vi "Write Device Metadata.vi"(0 "File Path":path, 11 "Error In":errorcluster) -> (4 "File Path (Dup)":path, 15 "Error Out":errorcluster)   [LabVIEW 2020]
uses:
  Hardware Configuration/Hardware Configuration Controls/Device Type.ctl
  Device Library/AOTFs/AOTF Controls/AOTF Actions.ctl
  Device Library/Cameras/Camera Controls/Generic Camera Actions.ctl
  Device Library/Lasers/Laser Controls/Laser Actions.ctl
  Device Library/Shutters/Shutter Controls/Shutter Actions.ctl
  Device Library/Stages/Stages Controls/Stage Actions.ctl
  Device Library/Filter Wheels/Polymorphic Filter Wheel Messenger/FW Get Position.vi
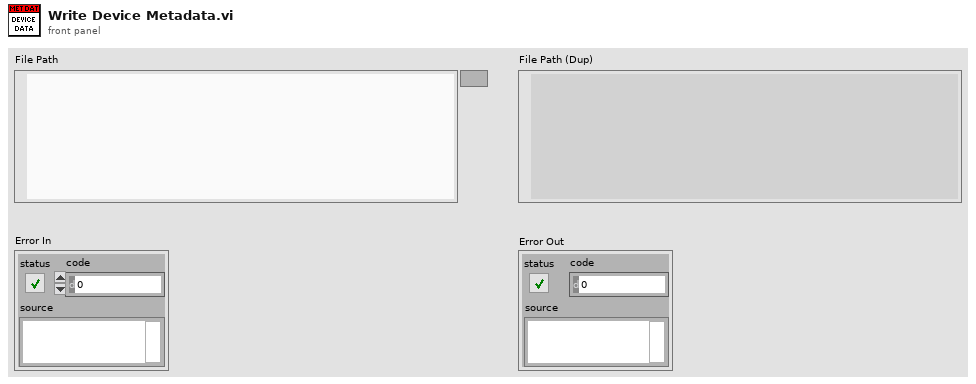
[diagram p1: front panel]
types:
  T1 = enum16{"open", "replace", "create", "open or create", "replace or create", "replace or create with confirmation"}
  T2 = typedef "Device Type.ctl" = enum16{"AOTF", "Camera", "Deformable Mirror", "Laser", "Microscope Base", "Shutter", "Stage", "Waveform", "FPGA", "Email", "Filter Wheel", "Spinning Disk"}
  T3 = typedef "Generic Camera Actions.ctl" = enum16{"Status", "Live Preview", "Capture", "Abort", "Set Exposure Time (s)", "Get Exposure Time (s)", "Record Settings", "Binning", "Set ROI", "Get ROI", "Defect Correction On?", "Cooler On?", "Fan On?", "Quit"}
  T4 = typedef "Laser Actions.ctl" = enum16{"Error Check", "Set On/Off", "Set Power", "Set Parameter", "Get Power", "Get Status", "Get Parameter", "Quit"}
  T5 = typedef "Shutter Actions.ctl" = enum16{"Open", "Close", "Toggle", "Status", "Quit"}
  T6 = typedef "Stage Actions.ctl" = enum16{"Get Position", "MVR", "MOVE", "HALT", "ONTARGET", "ERROR", "REFERENCE", "INIT", "VELOCITY", "STATUS", "EXIT", "HOME", "ZEROPOS", "NANOPOS", "ANALOG", "QUIT"}
  T7 = typedef "AOTF Actions.ctl" = enum16{"Error Check", "Blank", "Line On/Off", "Set Power", "Status", "Quit"}
  T8 = typedef "Laser Status.ctl" = enum16{"Warmup", "Ready", "Emission", "Tuning", "Error"}
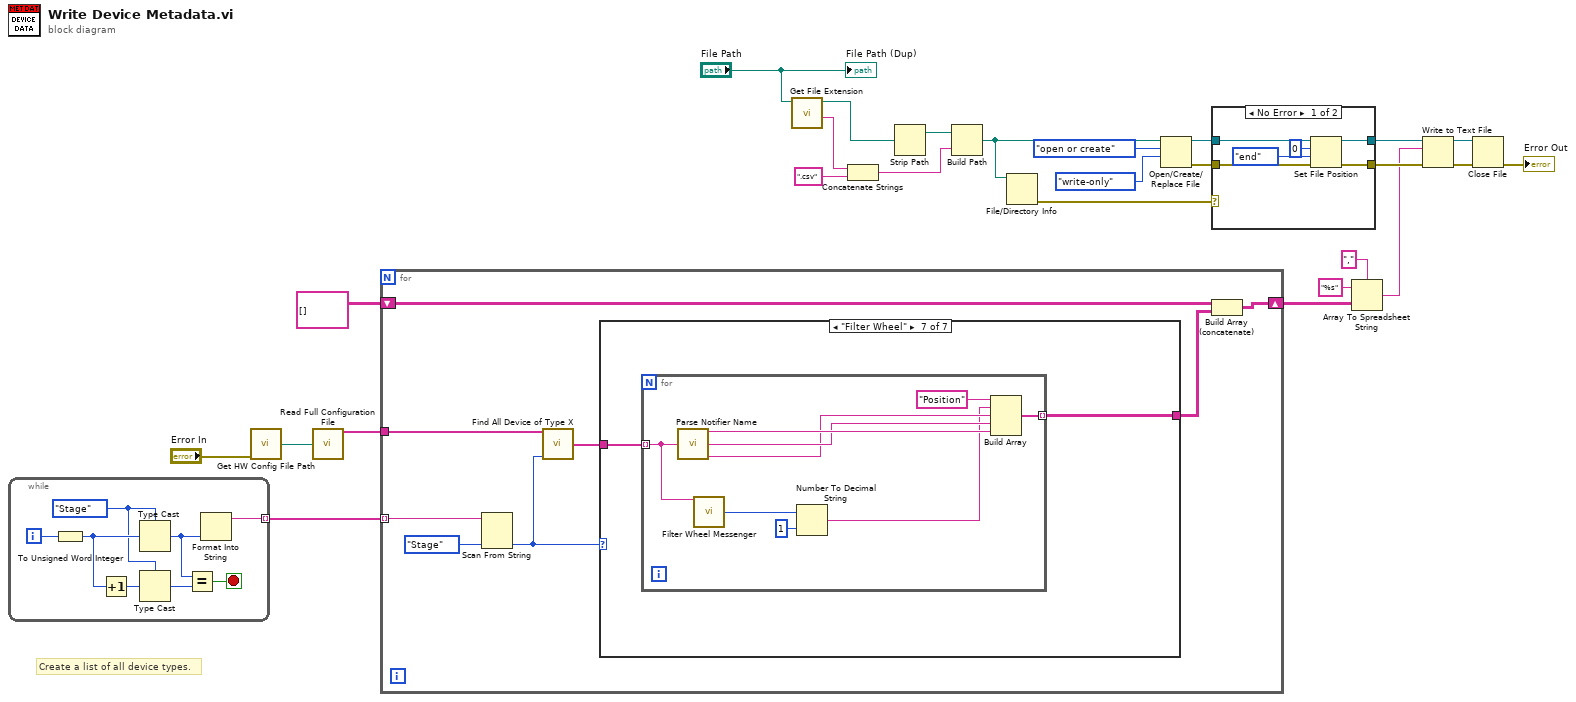
[diagram p0: block diagram]
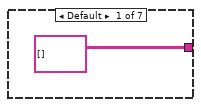
[diagram p3: hidden frame]
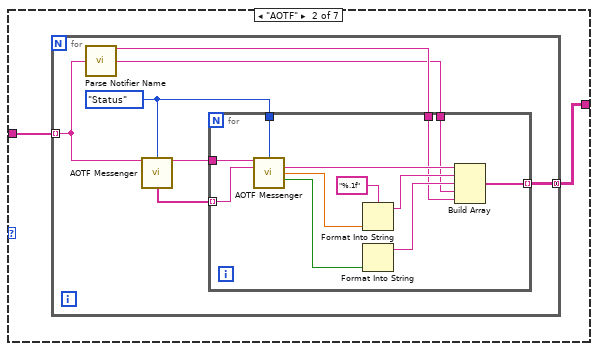
[diagram p4: hidden frame]
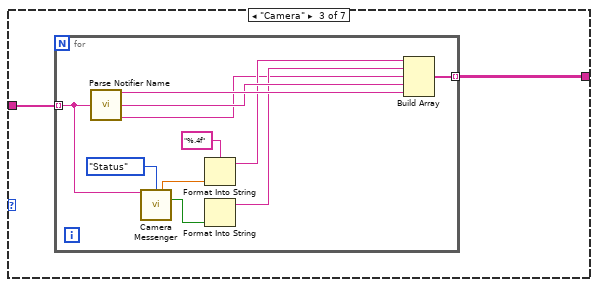
[diagram p5: hidden frame]
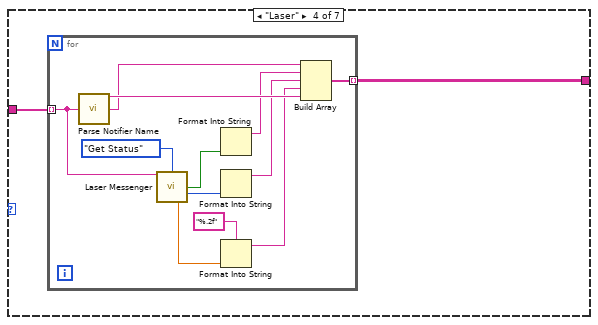
[diagram p6: hidden frame]
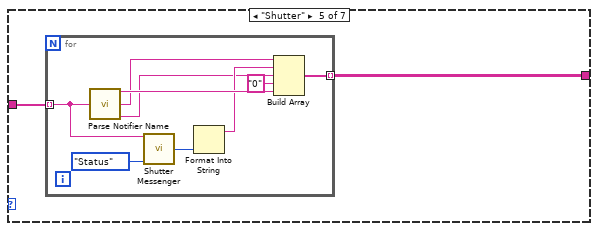
[diagram p7: hidden frame]
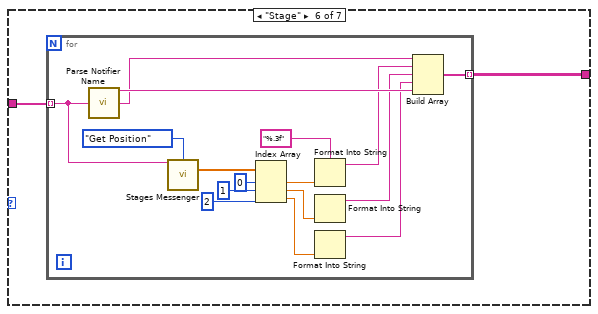
[diagram p8: hidden frame]
diagram:
  # "Create a list of all device types."
  n1 = while {
    tunnel: [w27] -> w26 mode=indexing
    i -> [w30]
    stop <- w29 stop-if-true
    w31 = Device_Type."Stage" ("Device Type")
    n2 = To Unsigned Word Integer(number=w30) -> (unsigned 16bit integer=w32:u16)
    n3 = Increment(x=w32) -> (x+1=w33:u16)
    n4 = Type Cast(type=w31, x=w32) -> (*(type *) &x=w28:T2)
    n5 = Type Cast(type=w31, x=w33) -> (*(type *) &x=w34:T2)
    n6 = Equal?(x=w28, y=w34) -> (x = y?=w29:bool)
    n7 = Format Into String(w28) -> (resulting string=w27:string)  [unwired: 3 in, 1 out]
  }
  n8 = call "Get HW Config File Path.vi"("Error"="Error In") -> ("File Path"=w25:path)  [unwired: 13 in, 1 out]
  n9 = call "Read Full Configuration File.vi"("Config File Path"=w25) -> ("Unique Notifier Names"=w24:string[])  [unwired: 11 in, 3 out]
  n10 = for {
    tunnel: w26 -> [w42] mode=indexing
    tunnel: w24 -> [w39]
    shift-right: [w36] -> w2
    shift-left: string[][] [] -> [w37]
    n11 = Scan From String(input string=w42, default 1=Device_Type."Stage" ("Device Type")) -> (output 1=w40:T2)  [unwired: 3 in, 3 out]
    n12 = call "Find All Device of Type X.vi"("Unique Notifier Names"=w39, "Device Type"=w40) -> ("Running Devices"=w38:string[])  [unwired: 12 in, 1 out]
    n13 = case shown="\"Filter Wheel\"" w40 {
      tunnel: w38 -> [_ w45 w66 w79 w93 w104 w122]
      tunnel: [string[][] [] w44 w65 w78 w92 w103 w121] -> w35
      frame Default {
      }
      frame "AOTF" {
        n14 = for {
          tunnel: w45 -> [w52] mode=indexing
          tunnel: [w46] -> w44 mode=concatenating
          w49 = AOTF_Actions."Status" ("AOTF Action")
          n15 = call "Parse Notifier Name.vi"("Notifier Name"=w52) -> ("Device Type"=w48:string, "Function"=w47:string)  [unwired: 12 in, 1 out]
          n16 = call "AOTF Messenger.vi"("AOTF Notifier Name"=w52, "AOTF Action"=w49) -> ("AOTF Notifier Name (Dup)"=w50:string, "Wavelengths (nm)"=w51:string[])  [unwired: 8 in, 4 out]
          n17 = for {
            tunnel: w51 -> [w63] mode=indexing
            tunnel: w50 -> [w64]
            tunnel: w49 -> [w62]
            tunnel: w48 -> [w55]
            tunnel: w47 -> [w54]
            tunnel: [w53] -> w46 mode=indexing
            n18 = call "AOTF Messenger.vi"("AOTF Notifier Name"=w64, "AOTF Action"=w62, "Wavelength (nm)"=w63) -> ("Wavelength (nm) Out"=w61:string, "Power (%) Out"=w59:dbl, "Line On/Off Out"=w57:bool)  [unwired: 7 in, 3 out]
            n19 = Format Into String(format string="%.1f", w59) -> (resulting string=w58:string)  [unwired: 2 in, 1 out]
            n20 = Format Into String(w57) -> (resulting string=w56:string)  [unwired: 3 in, 1 out]
            n21 = Build Array(w61, w58, w56, w54, w55) -> (w53:string[])
          }
        }
      }
      frame "Camera" {
        n22 = for {
          tunnel: w66 -> [w76] mode=indexing
          tunnel: [w67] -> w65 mode=indexing
          n23 = call "Parse Notifier Name.vi"("Notifier Name"=w76) -> ("Device Type"=w75:string, "Function"=w74:string, "Company"=w68:string)  [unwired: 12 in]
          n24 = call "Camera Messenger.vi"("Notifier Name"=w76, "General Camera Actions"=Generic_Camera_Actions."Status") -> ("Current Exposure Time (s)"=w72:dbl, "Running?"=w71:bool)  [unwired: 8 in, 4 out]
          n25 = Format Into String(format string="%.4f", w72) -> (resulting string=w70:string)  [unwired: 2 in, 1 out]
          n26 = Format Into String(w71) -> (resulting string=w69:string)  [unwired: 3 in, 1 out]
          n27 = Build Array(w70, w69, w68, w74, w75) -> (w67:string[])
        }
      }
      frame "Laser" {
        n28 = for {
          tunnel: w79 -> [w91] mode=indexing
          tunnel: [w80] -> w78 mode=indexing
          n29 = call "Parse Notifier Name.vi"("Notifier Name"=w91) -> ("Device Type"=w88:string, "Function"=w87:string)  [unwired: 12 in, 1 out]
          n30 = call "Laser Messenger.vi"("Notifier Name"=w91, "Action"=Laser_Actions."Get Status") -> ("Light Emission?"=w86:bool, "Laser Status"=w89:T8, "Power (mW)"=w85:dbl)  [unwired: 8 in, 3 out]
          n31 = Format Into String(w86) -> (resulting string=w83:string)  [unwired: 3 in, 1 out]
          n32 = Format Into String(w89) -> (resulting string=w82:string)  [unwired: 3 in, 1 out]
          n33 = Format Into String(format string="%.2f", w85) -> (resulting string=w81:string)  [unwired: 2 in, 1 out]
          n34 = Build Array(w87, w83, w82, w81, w88) -> (w80:string[])
        }
      }
      frame "Shutter" {
        n35 = for {
          tunnel: w93 -> [w102] mode=indexing
          tunnel: [w94] -> w92 mode=indexing
          n36 = call "Parse Notifier Name.vi"("Notifier Name"=w102) -> ("Device Type"=w100:string, "Function"=w99:string, "Company"=w96:string)  [unwired: 12 in]
          n37 = call "Shutter Messenger.vi"("Notifier Name"=w102, "Action"=Shutter_Actions."Status") -> ("Shutter Status"=w98:T5)  [unwired: 12 in, 1 out]
          n38 = Format Into String(w98) -> (resulting string=w97:string)  [unwired: 3 in, 1 out]
          n39 = Build Array(w99, w97, w96, "0" ("element"), w100) -> (w94:string[])
        }
      }
      frame "Stage" {
        n40 = for {
          tunnel: w104 -> [w120] mode=indexing
          tunnel: [w105] -> w103 mode=indexing
          n41 = call "Parse Notifier Name.vi"("Notifier Name"=w120) -> ("Device Type"=w118:string, "Function"=w117:string)  [unwired: 12 in, 1 out]
          n42 = call "Stages Messenger.vi"("Stage Notifier Name"=w120, "Actions"=Stage_Actions."Get Position") -> ("Positions"=w116:dbl[])  [unwired: 9 in, 4 out]
          n43 = Index Array(array=w116, index #1=0 ("index"), index #2=1 ("index"), index #3=2 ("index")) -> (element #1=w111:dbl, element #2=w109:dbl, element #3=w108:dbl)
          n44 = Format Into String(format string="%.3f", w111) -> (resulting string=w110:string)  [unwired: 2 in, 1 out]
          n45 = Format Into String(w109) -> (resulting string=w107:string)  [unwired: 3 in, 1 out]
          n46 = Format Into String(w108) -> (resulting string=w106:string)  [unwired: 3 in, 1 out]
          n47 = Build Array(w117, w110, w107, w106, w118) -> (w105:string[])
        }
      }
      frame "Filter Wheel" {
        n48 = for {
          tunnel: w122 -> [w127] mode=indexing
          tunnel: [w128] -> w121 mode=indexing
          n49 = call "Parse Notifier Name.vi"("Notifier Name"=w127) -> ("Device Type"=w131:string, "Function"=w130:string, "Company"=w129:string)  [unwired: 12 in]
          n50 = call-poly "Filter Wheel Messenger.vi"("Notifier Name In"=w127) -> ("Position"=w124:i32)  [unwired: 12 in, 2 out]
          n51 = Number To Decimal String(number=w124, width (-)=i16 1) -> (decimal integer string=w123:string)
          n52 = Build Array("Position" ("element"), w123, w129, w130, w131) -> (w128:string[])
        }
      }
    }
    n53 = Build Array (concatenate)(w37, w35) -> (w36:string[][])
  }
  n54 = call <vilib>:"Get File Extension.vi"("file"="File Path") -> ("filename without extension"=w11:string, "dup file"=w10:path)  [unwired: 6 in, 3 out]
  n55 = Concatenate Strings(w11, ".csv" ("string")) -> (w12:string)
  n56 = Strip Path(path=w10) -> (stripped path=w9:path)  [unwired: 1 out]
  n57 = Build Path(base path=w9, name or relative path=w12) -> (appended path=w13:path)
  n58 = File/Directory Info(path=w13) -> (error out=w14:errorcluster)  [unwired: 1 in, 6 out]
  n59 = Open/Create/Replace File(file path (use dialog)=w13, operation (0:open)=T1."open or create", access (0:read/write)=enum16{"read/write", "read-only", "write-only"}."write-only") -> (refnum out=w15:refnum<file>, error out=w16:errorcluster)  [unwired: 3 in, 1 out]
  n60 = case shown="No Error" w14 {
    tunnel: w15 -> [w137 w139]
    tunnel: w16 -> [w134 w138]
    tunnel: [w133 w139] -> w17
    tunnel: [w132 w138] -> w18
    frame No Error {
      n61 = Set File Position(offset (in bytes) (0)=i64 0, refnum=w137, from (0:start)=enum16{"start", "end", "current"}."end", error in=w134) -> (refnum out=w133:refnum<file>, error out=w132:errorcluster)
    }
    frame Error {
    }
  }
  n62 = Array To Spreadsheet String(delimiter (Tab)=",", array=w2, 3:"%s" ("format string")) -> (spreadsheet string=w5:string)
  n63 = Write to Text File(file (use dialog)=w17, text=w5, error in=w18) -> (refnum out=w19:refnum<file>, error out=w20:errorcluster)  [unwired: 1 in, 1 out]
  n64 = Close File(refnum=w19, error in=w20) -> (error out=→"Error Out":errorcluster)  [unwired: 1 out]
  "File Path (Dup)" <- "File Path"
